vi "ADC Simulated.vi"(11 "Command to Send":string="SRC012;") -> (2 "ADC":dbl, 3 "Puerto":string)   [LabVIEW 2020, in "UI Actor.lvlib" / "UI Actor.lvclass"]
uses:
  UI Actor.lvclass
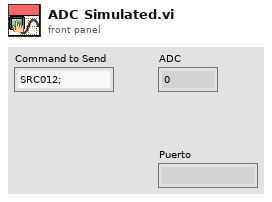
[diagram p1: front panel]
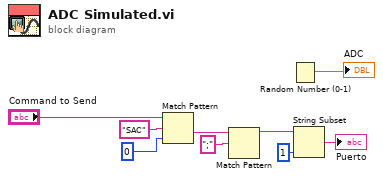
[diagram p0: block diagram]
diagram:
  n1 = Match Pattern(string="Command to Send", regular expression="SAC" ("string"), offset (0)=0) -> (after substring=w5:string)  [unwired: 3 out]
  n2 = Match Pattern(string=w5, regular expression=";") -> (before substring=w1:string)  [unwired: 1 in, 3 out]
  n3 = Random Number (0-1)() -> (number: 0 to 1=→"ADC":dbl)
  n4 = String Subset(string=w1, length (rest)=1 ("length (rest)")) -> (substring=→"Puerto":string)  [unwired: 1 in]
